vi "Global Variable Control (Front Panel Design of Global Variable).vi"() -> ()   [LabVIEW 2016]
panel:
  in  "Boolean":bool
  in  "Slide":dbl(slide) scale=0.0..100.0
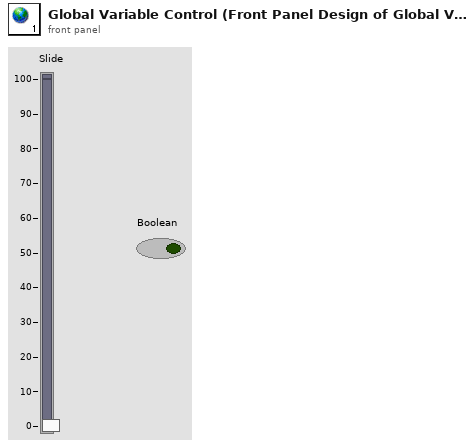
[diagram p1: front panel]
diagram:
